vi "test_Series Actor PID Simulated Scope Simualted FGen.vi"(8 "Error In":errorcluster) -> (0 "Error Out":errorcluster)   [LabVIEW 2023]
uses:
  Series/Series Base/Series Base.lvclass
  Series/Series Actor/Series Actor/Series Actor.lvclass
  Scope/Virtual Scopes/Virt Voltage Reader/Virt Voltage Reader.lvclass
  FGen/Virtual FGens/Virt Voltage Generator/Virt Voltage Generator.lvclass
  FGen/FGen Simulated/Configurations/Generate DC CFG/Generate DC CFG.lvclass
  Scope/Scope Simulated/Configurations/Fetch Waveforms CFG/Fetch Waveforms CFG.lvclass
  Sample Tasks/Sample PID Light/Sample PID Light.lvclass
  Sample Tasks/Sample PID Flow/Sample PID Flow.lvclass
  Sample Series/Sample Photosensor PID Flowsensor PID/Sample Photosensor PID Flowsensor PID/Sample Photosensor PID Flowsensor PID.lvclass
  DIO/DIO DAQmx Simulated CFGs/CO DAQmx PWM Fixed Freq CFG/CO DAQmx PWM Fixed Freq CFG.lvclass
  DIO/Virtual DIO/Virt PWM Fixed Freq Generator/Virt DAQmx Fixed Freq PWM Generator.lvclass
  Series/Series Actor/Series Actor/Series Actor.lvclass/Series Actor.ctl
  1fb8c4b3-f1dd-453f-83af-f5a0d3a15630.vi
  <vilib>/JDP Science/JSONtext/Find Item.vi
  <vilib>/JDP Science/JSONtext/Next JSON Value.vi
  <vilib>/JDP Science/JSONtext/String Subset.vi
  <vilib>/JDP Science/JSONtext/Parsing/Advance past next JSON Value (inlined COPY).vi
  <vilib>/JDP Science/JSONtext/Parsing/Advance past whitespace.vi
  <vilib>/JDP Science/JSONtext/Parsing/Advance past String.vi
  <vilib>/JDP Science/JSONtext/Parsing/Advance past Number.vi
  <vilib>/JDP Science/JSONtext/Parsing/Advance past Line Ending.vi
  <vilib>/JDP Science/JSONtext/Parsing/Parse Full Path or Item Name.vi
  <vilib>/JDP Science/JSONtext/Parsing/Advance past Array.vi
  <vilib>/JDP Science/JSONtext/Parsing/Advance past Object.vi
  <vilib>/JDP Science/JSONtext/support/Error Cluster From Code.vi
  <vilib>/JDP Science/JSONtext/Offset/Find Item Locations by Path.vi
  <vilib>/JDP Science/JSONtext/JSON text to Variant.vi
  <vilib>/JDP Science/JSONtext/LVClass Serializer/JSONtext LVClass Serializer.lvclass
  <vilib>/ActorFramework/Actor/Actor.lvclass
panel:
  in  "Stop":bool
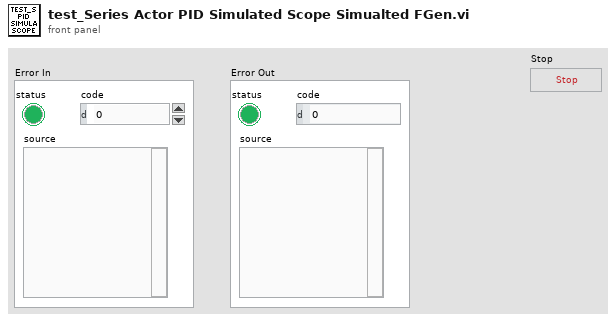
[diagram p1: front panel]
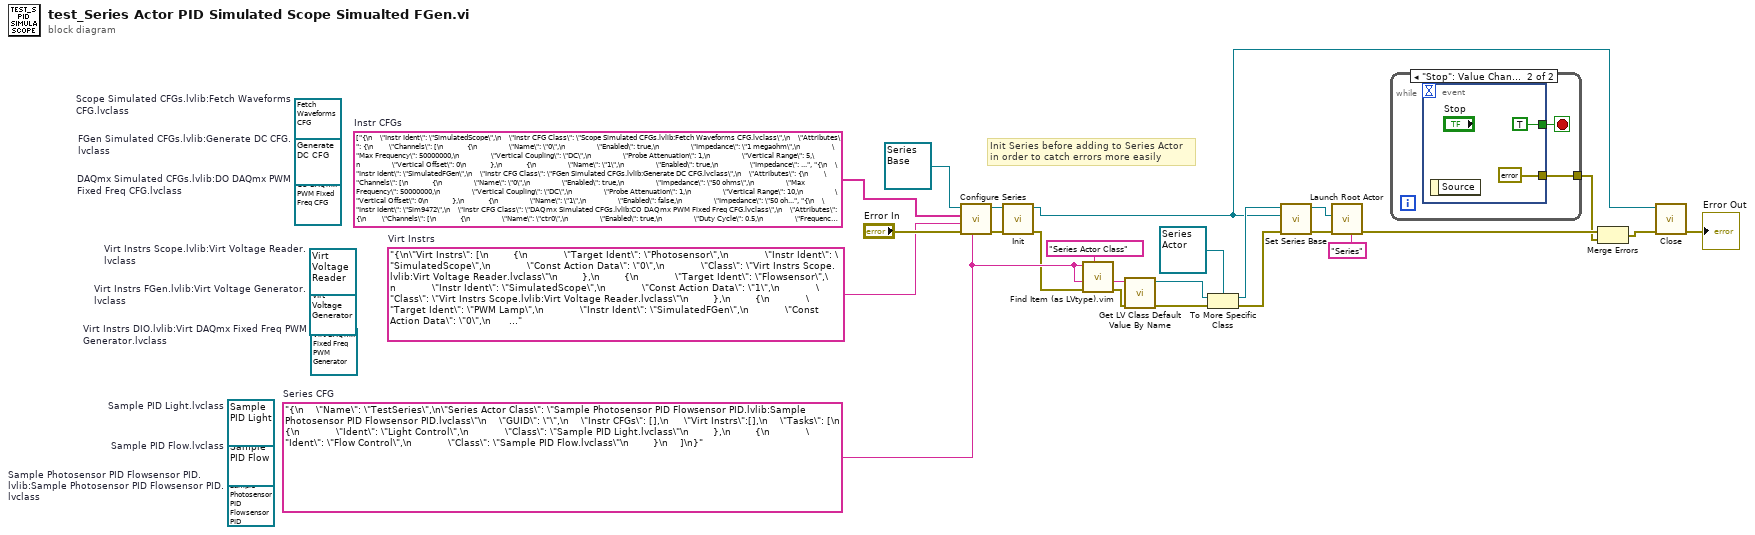
[diagram p0: block diagram]
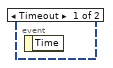
[diagram p2: hidden frame]
diagram:
  (unwired) refnum<class "Virt DAQmx Fixed Freq PWM Generator.lvclass"> refnum  # Virt Instrs DIO.lvlib:Virt DAQmx Fixed Freq PWM Generator.lvclass
  (unwired) refnum<class "CO DAQmx PWM Fixed Freq CFG.lvclass"> refnum  # DAQmx Simulated CFGs.lvlib:DO DAQmx PWM Fixed Freq CFG.lvclass
  (unwired) refnum<class "Sample Photosensor PID Flowsensor PID.lvclass"> refnum  # Sample Photosensor PID Flowsensor PID.lvlib:Sample Photosensor PID Flowsensor PID.lvclass
  (unwired) refnum<class "Sample PID Flow.lvclass"> refnum  # Sample PID Flow.lvclass
  (unwired) refnum<class "Sample PID Light.lvclass"> refnum  # Sample PID Light.lvclass
  (unwired) refnum<class "Fetch Waveforms CFG.lvclass"> refnum  # Scope Simulated CFGs.lvlib:Fetch Waveforms CFG.lvclass
  (unwired) refnum<class "Generate DC CFG.lvclass"> refnum  # FGen Simulated CFGs.lvlib:Generate DC CFG.lvclass
  (unwired) refnum<class "Virt Voltage Generator.lvclass"> refnum  # Virt Instrs FGen.lvlib:Virt Voltage Generator.lvclass
  (unwired) refnum<class "Virt Voltage Reader.lvclass"> refnum  # Virt Instrs Scope.lvlib:Virt Voltage Reader.lvclass
  w18 = "{\n\"Virt Instrs\": [\n        {\n            \"Target Ident\": \"Photosensor\",\n            \"Instr Ident\": \"SimulatedScope\",\n            \"Const Action Data\": \"0\",\n            \"Class\": \"Virt Instrs Scope.lvlib:Virt Voltage Reader.lvclass\"\n        },\n        {\n            \"Target Ident\": \"Flowsensor\",\n            \"Instr Ident\": \"SimulatedScope\",\n            \"Const Action Data\": \"1\",\n            \"Class\": \"Virt Instrs Scope.lvlib:Virt Voltage Reader.lvclass\"\n        },\n        {\n            \"Target Ident\": \"PWM Lamp\",\n            \"Instr Ident\": \"SimulatedFGen\",\n            \"Const Action Data\": \"0\",\n            \"Class\": \"Virt Instrs FGen.lvlib:Virt Voltage Generator.lvclass\"\n        },\n        {\n            \"Target Ident\": \"PWM Flow\",\n            \"Instr Ident\": \"Sim9472\",\n            \"Const Action Data\": \"0\",\n            \"Class\": \"Virt Instrs DIO.lvlib:Virt DAQmx Fixed Freq PWM Generator.lvclass\"\n        }\n    ]\n}"  # Virt Instrs
  w17 = string[] ["{\n    \"Instr Ident\": \"SimulatedScope\",\n    \"Instr CFG Class\": \"Scope Simulated CFGs.lvlib:Fetch Waveforms CFG.lvclass\",\n    \"Attributes\": {\n        \"Channels\": [\n            {\n                \"Name\": \"0\",\n                \"Enabled\": true,\n                \"Impedance\": \"1 megaohm\",\n                \"Max Frequency\": 50000000,\n                \"Vertical Coupling\": \"DC\",\n                \"Probe Attenuation\": 1,\n                \"Vertical Range\": 5,\n                \"Vertical Offset\": 0\n            },\n            {\n                \"Name\": \"1\",\n                \"Enabled\": true,\n                \"Impedance\": \"50 ohms\",\n                \"Max Frequency\": 50000000,\n                \"Vertical Coupling\": \"DC\",\n                \"Probe Attenuation\": 1,\n                \"Vertical Range\": 5,\n                \"Vertical Offset\": 0\n            },\n            {\n                \"Name\": \"2\",\n                \"Enabled\": false,\n                \"Impedance\": \"50 ohms\",\n                \"Max Frequency\": 50000000,\n                \"Vertical Coupling\": \"DC\",\n                \"Probe Attenuation\": 1,\n                \"Vertical Range\": 5,\n                \"Vertical Offset\": 0\n            },\n            {\n                \"Name\": \"3\",\n                \"Enabled\": false,\n                \"Impedance\": \"50 ohms\",\n                \"Max Frequency\": 50000000,\n                \"Vertical Coupling\": \"DC\",\n                \"Probe Attenuation\": 1,\n                \"Vertical Range\": 1.4,\n                \"Vertical Offset\": 0\n            },\n            {\n                \"Name\": \"4\",\n                \"Enabled\": false,\n                \"Impedance\": \"50 ohms\",\n                \"Max Frequency\": 50000000,\n                \"Vertical Coupling\": \"DC\",\n                \"Probe Attenuation\": 1,\n                \"Vertical Range\": 5,\n                \"Vertical Offset\": 0\n            },\n            {\n                \"Name\": \"5\",\n                \"Enabled\": false,\n                \"Impedance\": \"50 ohms\",\n                \"Max Frequency\": 50000000,\n                \"Vertical Coupling\": \"DC\",\n                \"Probe Attenuation\": 1,\n                \"Vertical Range\": 5,\n                \"Vertical Offset\": 0\n            },\n            {\n                \"Name\": \"6\",\n                \"Enabled\": false,\n                \"Impedance\": \"50 ohms\",\n                \"Max Frequency\": 50000000,\n                \"Vertical Coupling\": \"DC\",\n                \"Probe Attenuation\": 1,\n                \"Vertical Range\": 5,\n                \"Vertical Offset\": 0\n            },\n            {\n                \"Name\": \"7\",\n                \"Enabled\": false,\n                \"Impedance\": \"50 ohms\",\n                \"Max Frequency\": 50000000,\n                \"Vertical Coupling\": \"DC\",\n                \"Probe Attenuation\": 1,\n                \"Vertical Range\": 5,\n                \"Vertical Offset\": 0\n            }\n        ],\n        \"Horizontal\": {\n            \"Enforce Realtime\": true,\n            \"Number of Records\": 1,\n            \"Min Sample Rate\": 100000,\n            \"Reference Position\": 50,\n            \"Min Record Length\": 1000\n        },\n        \"Acquire\": {\n            \"Type\": \"Normal\",\n            \"NumSamples\": 1000,\n            \"Fetch Relative To\": \"Read Pointer\"\n        },\n        \"Export Signal\": {\n            \"Signal Identifier\": \"None\",\n            \"Signal\": \"None\",\n            \"Output Terminal\": \"None\"\n        },\n        \"Trigger\": {\n            \"Type\": \"Immediate\",\n            \"Slope\": \"Positive\",\n            \"Source\": \"RTSI 0\",\n            \"Holdoff\": 0,\n            \"Delay\": 0\n        }\n    }\n}", "{\n    \"Instr Ident\": \"SimulatedFGen\",\n    \"Instr CFG Class\": \"FGen Simulated CFGs.lvlib:Generate DC CFG.lvclass\",\n    \"Attributes\": {\n        \"Channels\": [\n            {\n                \"Name\": \"0\",\n                \"Enabled\": true,\n                \"Impedance\": \"50 ohms\",\n                \"Max Frequency\": 50000000,\n                \"Vertical Coupling\": \"DC\",\n                \"Probe Attenuation\": 1,\n                \"Vertical Range\": 10,\n                \"Vertical Offset\": 0\n            },\n            {\n                \"Name\": \"1\",\n                \"Enabled\": false,\n                \"Impedance\": \"50 ohms\",\n                \"Max Frequency\": 50000000,\n                \"Vertical Coupling\": \"DC\",\n                \"Probe Attenuation\": 1,\n                \"Vertical Range\": 0.2,\n                \"Vertical Offset\": 0\n            }\n        ],\n        \"Horizontal\": {\n            \"Enforce Realtime\": true,\n            \"Number of Records\": 1,\n            \"Min Sample Rate\": 100000,\n            \"Reference Position\": 50,\n            \"Min Record Length\": 1000\n        },\n        \"Acquire\": {\n            \"Type\": \"Normal\"\n        },\n        \"Export Signal\": {\n            \"Enabled\": false,\n            \"Signal Identifier\": \"None\",\n            \"Signal\": \"None\",\n            \"Output Terminal\": \"None\"\n        },\n        \"Trigger\": {\n            \"Type\": \"Digital\",\n            \"Source\": \"RTSI 0\",\n            \"Holdoff\": 0,\n            \"Delay\": 0\n        }\n    }\n}", "{\n    \"Instr Ident\": \"Sim9472\",\n    \"Instr CFG Class\": \"DAQmx Simulated CFGs.lvlib:CO DAQmx PWM Fixed Freq CFG.lvclass\",\n    \"Attributes\": {\n        \"Channels\": [\n            {\n                \"Name\": \"ctr0\",\n                \"Enabled\": true,\n                \"Duty Cycle\": 0.5,\n                \"Frequency\": 600,\n                \"Units\": \"Hz\",\n                \"Idle State\": \"Low\",\n                \"Initial Delay\": 0\n            },\n            {\n                \"Name\": \"ctr1\",\n                \"Enabled\": false,\n                \"Duty Cycle\": 0.5,\n                \"Frequency\": 1,\n                \"Units\": \"Hz\",\n                \"Idle State\": \"Low\",\n                \"Initial Delay\": 0\n            },\n            {\n                \"Name\": \"ctr2\",\n                \"Enabled\": false,\n                \"Duty Cycle\": 0.5,\n                \"Frequency\": 1,\n                \"Units\": \"Hz\",\n                \"Idle State\": \"Low\",\n                \"Initial Delay\": 0\n            },\n            {\n                \"Name\": \"ctr3\",\n                \"Enabled\": false,\n                \"Duty Cycle\": 0.5,\n                \"Frequency\": 1,\n                \"Units\": \"Hz\",\n                \"Idle State\": \"Low\",\n                \"Initial Delay\": 0\n            }\n        ],\n        \"Timing\": {\n            \"Samples per Channel\": 1000,\n            \"Sample Mode\": \"Continuous Samples\",\n            \"Sample Rate\": 0,\n            \"Sample Clock Source\": \"Implicit\",\n            \"Active Edge\": \"Rising\"\n        },\n        \"Trigger\": {\n            \"Trigger Type\": \"No Trigger\"\n        }\n    }\n}"]  # Instr CFGs
  w12 = "{\n    \"Name\": \"TestSeries\",\n\"Series Actor Class\": \"Sample Photosensor PID Flowsensor PID.lvlib:Sample Photosensor PID Flowsensor PID.lvclass\"\n    \"GUID\": \"\",\n    \"Instr CFGs\": [],\n     \"Virt Instrs\":[],\n    \"Tasks\": [\n        {\n            \"Ident\": \"Light Control\",\n            \"Class\": \"Sample PID Light.lvclass\"\n        },\n        {\n            \"Ident\": \"Flow Control\",\n            \"Class\": \"Sample PID Flow.lvclass\"\n        }\n    ]\n}"  # Series CFG
  # "Init Series before adding to Series Actor\nin order to catch errors more easily"
  n1 = call "Configure Series.vi"("Series CFG"=w12, "error in (no error)"="Error In", "Virt Instrs CFG"=w18, "Instr CFGs"=w17, "HAL GOOP4:Series Base in"=refnum<class "Series Base.lvclass"> refnum ("HAL GOOP4.lvlib:Study Base.lvclass")) -> ("error out"=w22:errorcluster, "HAL GOOP4:Series Base out"=w20:refnum<class "Series Base.lvclass">)  [unwired: 5 in]
  n2 = call-dynamic "Init.vi"("error in"=w22, "HAL GOOP4:Series Base in"=w20) -> ("error out"=w9:errorcluster, "HAL GOOP4:Series Base out"=w3:refnum<class "Series Base.lvclass">)  [unwired: 8 in]
  n3 = call "Find Item (as LVtype).vim"("$Path or Item Name"="Series Actor Class", "error in (no error)"=w9, "Data Type and Default Value"=w12, "JSON"=w12) -> ("error out"=w10:errorcluster, "Data"=w11:string)  [unwired: 4 in, 2 out]
  n4 = call <vilib>:"Get LV Class Default Value By Name.vi"("error in (no error)"=w10, "class name"=w11) -> ("error out"=w15:errorcluster, "object"=w14:refnum<class>)  [unwired: 8 in]
  n5 = To More Specific Class(target class=refnum<class "Series Actor.lvclass"> refnum ("Series Actor.lvlib:Series Actor.lvclass"), reference=w14, error in=w15) -> (specific class reference=w6:refnum<class "Series Actor.lvclass">, error out=w8:errorcluster)
  n6 = call "Set Series Base.vi"("error in (no error)"=w8, "Series Base"=w3, "Series Actor in"=w6) -> ("error out"=w16:errorcluster, "Series Actor out"=w23:refnum<class "Series Actor.lvclass">)  [unwired: 7 in]
  n7 = call <vilib>:"Launch Root Actor.vi"("Debug Alias"="Series", "error in (no error)"=w16, "Actor"=w23) -> ("error out"=w5:errorcluster)  [unwired: 7 in, 1 out]
  n8 = while {
    tunnel: [w25] -> w1
    stop <- w26 stop-if-true
    n9 = event shown="[1] \"Stop\": Value Change" {
      selector: _ -> [_ _]
      dyn-events: _ -> [_ _]
      timeout: _ -> [_ _]
      tunnel: [_ TRUE] -> w26
      tunnel: [_ errorcluster {"status"=FALSE, "code"=0, "source"=""} ("error constant")] -> w25
      event Timeout {
        n10 = event-data() -> ()  [unwired: 1 in, 1 out]
      }
      event "Stop": Value Change {
        n11 = event-data() -> ()  [unwired: 1 in, 1 out]
      }
    }
  }
  n12 = Merge Errors(w5, w1) -> (w2:errorcluster)
  n13 = call-dynamic "Close.vi"("error in"=w2, "Series Base in"=w3) -> ("error out"=→"Error Out":errorcluster)  [unwired: 8 in, 1 out]
